vi "2nd screen effect (SubVI).vi"(1 "MeasVelScrnSet 2":sgl, 2 "MeasVelScrnSet 1":sgl, 3 "2nd Screen ref":refnum<vi>) -> (0 "MeasVelOut":sgl)   [LabVIEW 2015]
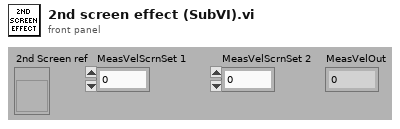
[diagram p1: front panel]
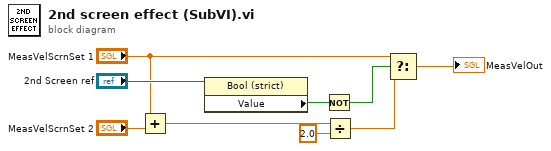
[diagram p0: block diagram]
diagram:
  n1 = Add(x="MeasVelScrnSet 1", y="MeasVelScrnSet 2") -> (x+y=w1:sgl)
  n2 = property class="Bool (strict)"(reference="2nd Screen ref") -> ("Value"=w6:bool)  [unwired: 1 in, 2 out]
  n3 = Not(x=w6) -> (.not. x?=w9:bool)
  n4 = Divide(x=w1, y=sgl 2.0) -> (x/y=w7:sgl)
  n5 = Select(t="MeasVelScrnSet 1", s=w9, f=w7) -> (s? t:f=→"MeasVelOut":sgl)
